vi "Parse Catagories.vi"(8 "error in (no error)":errorcluster {"code" format="Error %.0f"}, 10 "File Paths":path[](array[path]), 11 "VIDoc Parser In":refnum<class "VIDoc Parser.lvclass">) -> (0 "error out":errorcluster {"code" format="Error %.0f"}, 3 "VIDoc Parser Out":refnum<class "VIDoc Parser.lvclass">)   [LabVIEW 2023, in "VIDoc Parsing.lvlib" / "VIDoc Parser.lvclass"]
uses:
  VIDoc Parser.lvclass
  VIDoc Parser.lvclass/VIDoc Parser.ctl
  UI Interaction/UI Interaction.lvclass
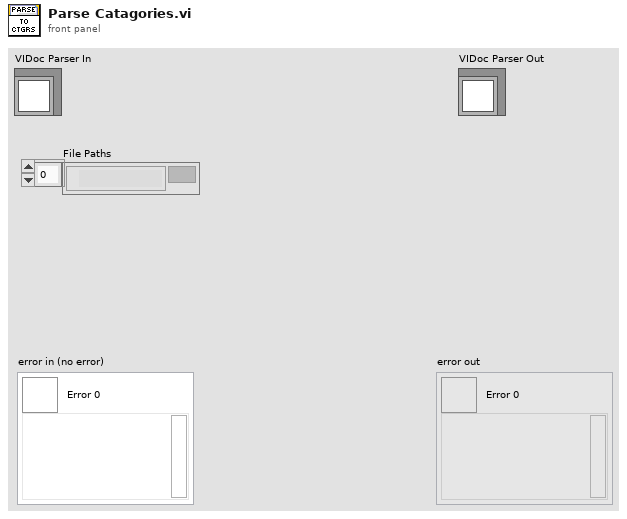
[diagram p1: front panel]
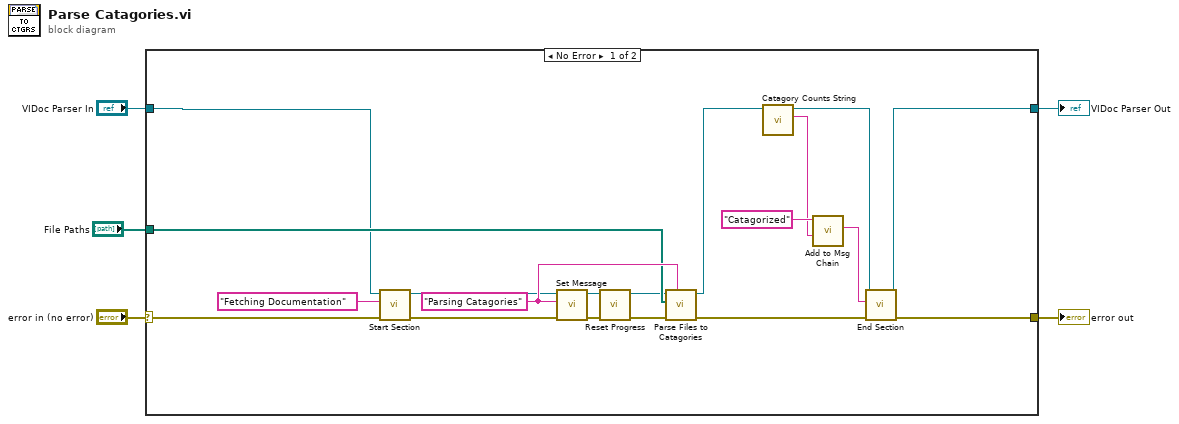
[diagram p0: block diagram]
diagram:
  n1 = case shown="No Error" "error in (no error)" {
    selector: "error in (no error)" -> [w22 w26]
    tunnel: [w19 w26] -> w4
    tunnel: [w6 w25] -> w2
    tunnel: "VIDoc Parser In" -> [w8 w25]
    tunnel: "File Paths" -> [w12 _]
    frame No Error {
      w13 = "Parsing Catagories" ("Message")
      n2 = call "Start Section.vi"("error in (no error)"=w22, "Section"="Fetching Documentation" ("format string"), "VIDoc Parser In"=w8) -> ("error out"=w21:errorcluster, "VIDoc Parser Out"=w10:refnum<class "VIDoc Parser.lvclass">)  [unwired: 7 in]
      n3 = call "Set Message.vi"("error in (no error)"=w21, "Message"=w13, "VIDoc Parser In"=w10) -> ("error out"=w23:errorcluster, "VIDoc Parser Out"=w24:refnum<class "VIDoc Parser.lvclass">)  [unwired: 7 in]
      n4 = call "Reset Progress.vi"("error in (no error)"=w23, "VIDoc Parser In"=w24) -> ("error out"=w15:errorcluster, "VIDoc Parser Out"=w9:refnum<class "VIDoc Parser.lvclass">)  [unwired: 8 in]
      n5 = call "Parse Files to Catagories.vi"("Message Chain"=w13, "Error in"=w15, "File Paths"=w12, "VIDoc Parser In"=w9) -> ("Error out"=w11:errorcluster, "VIDoc Parser Out"=w14:refnum<class "VIDoc Parser.lvclass">)  [unwired: 5 in, 1 out]
      n6 = call "Catagory Counts String.vi"("VIDoc Parser In"=w14) -> ("Catagory Counts"=w17:string, "VIDoc Parser Out"=w7:refnum<class "VIDoc Parser.lvclass">)  [unwired: 8 in, 1 out]
      n7 = call "Add to Msg Chain.vi"("New"=w17, "Msg Chain in"="Catagorized" ("format string")) -> ("Msg Chain out"=w16:string)  [unwired: 9 in]
      n8 = call "End Section.vi"("error in (no error)"=w11, "Section"=w16, "VIDoc Parser In"=w7) -> ("error out"=w19:errorcluster, "VIDoc Parser Out"=w6:refnum<class "VIDoc Parser.lvclass">)  [unwired: 7 in]
    }
    frame Error {
    }
  }
  "error out" <- w4
  "VIDoc Parser Out" <- w2
